vi "Add dark EQE measurement to queue.vi"(11 "Cell settings cluster":T2) -> (3 "Light/dark array":T1(array[cluster]))   [LabVIEW 2016]
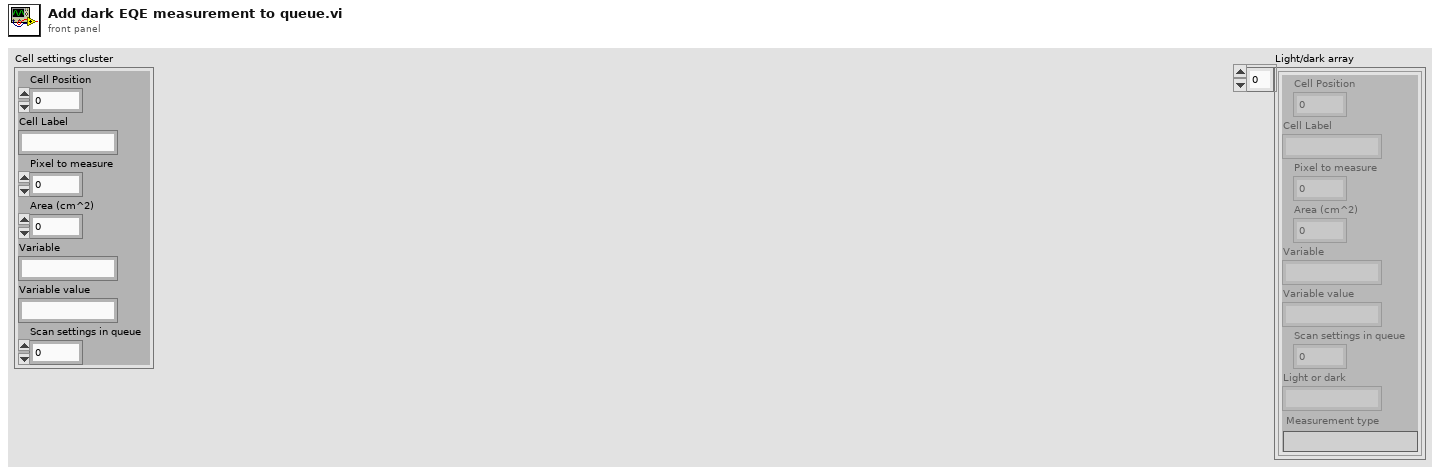
[diagram p1: front panel]
types:
  T1 = cluster{"Cell Position":i32, "Cell Label":string, "Pixel to measure":u16, "Area (cm^2)":dbl, "Variable":string, "Variable value":string, "Scan settings in queue":u16, "Light or dark":string, "Measurement type":string}[]
  T2 = cluster{"Cell Position":i32, "Cell Label":string, "Pixel to measure":u16, "Area (cm^2)":dbl, "Variable":string, "Variable value":string, "Scan settings in queue":u16}
  T3 = cluster{"Cell Position":i32, "Cell Label":string, "Pixel to measure":u16, "Area (cm^2)":dbl, "Variable":string, "Variable value":string, "Scan settings in queue":u16, "Light or dark":string, "Measurement type":string}
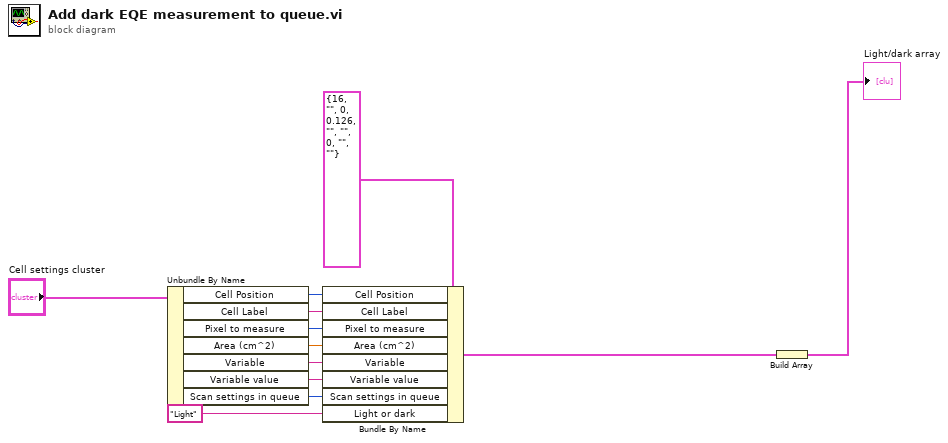
[diagram p0: block diagram]
diagram:
  n1 = Unbundle By Name("Cell settings cluster") -> ("Cell Position"=w4:i32, "Cell Label"=w5:string, "Pixel to measure"=w6:u16, "Area (cm^2)"=w7:dbl, "Variable"=w8:string, "Variable value"=w9:string, "Scan settings in queue"=w12:u16)
  n2 = Bundle By Name(cluster=T3 {"Cell Position"=16, "Cell Label"="", "Pixel to measure"=0, "Area (cm^2)"=0.126, "Variable"="", "Variable value"="", "Scan settings in queue"=0, "Light or dark"="", "Measurement type"=""} ("System Cluster"), "Cell Position"=w4, "Cell Label"=w5, "Pixel to measure"=w6, "Area (cm^2)"=w7, "Variable"=w8, "Variable value"=w9, "Scan settings in queue"=w12, "Light or dark"="Light") -> (w2:T3)
  n3 = Build Array(w2) -> (→"Light/dark array":T1)
